vi "CRYInitialize Menu State.vi"(8 "sAction":string, 11 "Is Disable?":bool) -> ()   [LabVIEW 2013]
uses:
  SubVI/CRYMain Sub Window Global.vi
  CRYMainGlobal.vi
  CRYSystem/Task Sequence/CRYProject Run Control Global.vi
  CRYSystem/Calibration/SubVI/CRYCal Global.vi
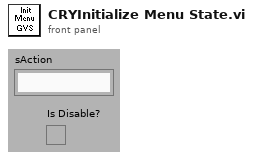
[diagram p1: front panel]
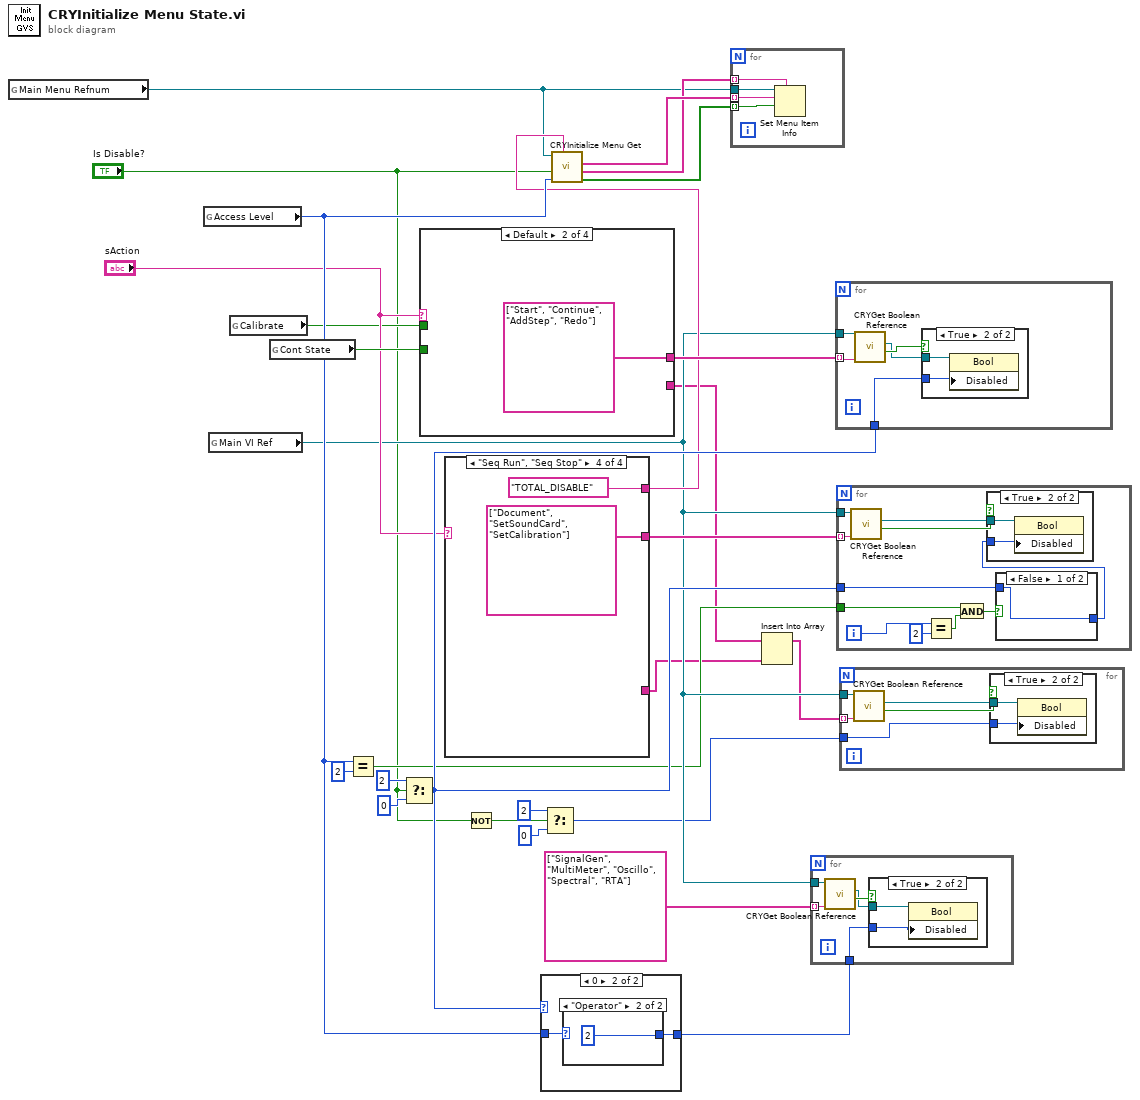
[diagram p0: block diagram]
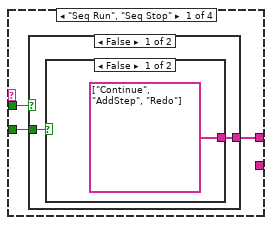
[diagram p3: hidden frame]
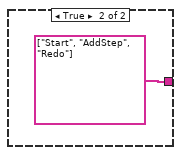
[diagram p4: hidden frame]
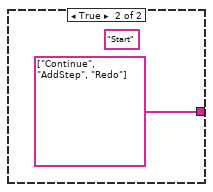
[diagram p5: hidden frame]
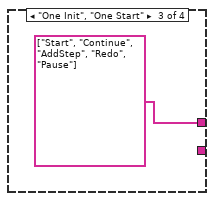
[diagram p6: hidden frame]
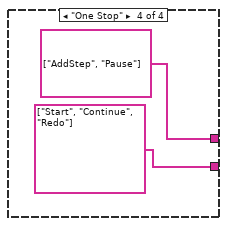
[diagram p7: hidden frame]
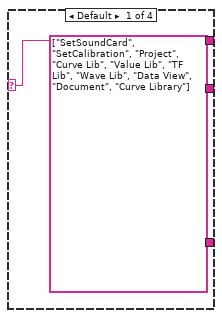
[diagram p8: hidden frame]
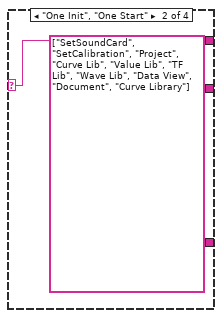
[diagram p9: hidden frame]
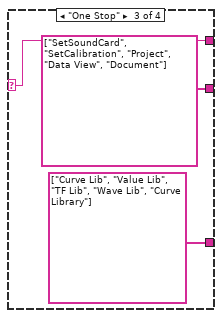
[diagram p10: hidden frame]
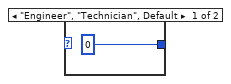
[diagram p12: hidden frame]
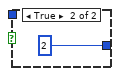
[diagram p14: hidden frame]
diagram:
  n1 = global read "CRYMain Sub Window Global.vi" "Main Menu Refnum"() -> (w1:refnum<k9>)
  n2 = global read "CRYMainGlobal.vi" "Access Level"() -> (w17:enum16{"Engineer", "Technician", "Operator"})
  n3 = global read "CRYMain Sub Window Global.vi" "Main VI Ref"() -> (w11:refnum<vi>)
  n4 = global read "CRYCal Global.vi" "Calibrate"() -> (w12:bool)
  n5 = global read "CRYProject Run Control Global.vi" "Cont State"() -> (w14:bool)
  n6 = Equal?(x=w17, y=u16 2) -> (x = y?=w10:bool)
  n7 = Select(t=u8 2 ("Disabled"), s="Is Disable?", f=u8 0) -> (s? t:f=w23:u8)
  n8 = case shown="Default" "sAction" {
    tunnel: [w29 string[] ["Start", "Continue", "AddStep", "Redo"] ("Array") string[] ["Start", "Continue", "AddStep", "Redo", "Pause"] ("Array") string[] ["AddStep", "Pause"] ("Array")] -> w26
    tunnel: w14 -> [w30 _ _ _]
    tunnel: w12 -> [w28 _ _ _]
    tunnel: [_ _ _ string[] ["Start", "Continue", "Redo"] ("Array")] -> w4
    frame "Seq Run", "Seq Stop" {
      n9 = case shown="False" w28 {
        tunnel: w30 -> [w32 _]
        tunnel: [w31 string[] ["Continue", "AddStep", "Redo"] ("Array")] -> w29
        frame False {
          n10 = case shown="False" w32 {
            tunnel: [string[] ["Continue", "AddStep", "Redo"] ("Array") string[] ["Start", "AddStep", "Redo"] ("Array")] -> w31
            frame False {
            }
            frame True {
            }
          }
        }
        frame True {
          (unwired) "Start"
        }
      }
    }
    frame Default {
    }
    frame "One Init", "One Start" {
    }
    frame "One Stop" {
    }
  }
  n11 = case shown="\"Seq Run\", \"Seq Stop\"" "sAction" {
    selector: "sAction" -> [w40 w42 w45 _]
    tunnel: [string[] ["SetSoundCard", "SetCalibration", "Project", "Curve Lib", "Value Lib", "TF Lib", "Wave Lib", "Data View", "Document", "Curve Library"] ("Array") string[] ["SetSoundCard", "SetCalibration", "Project", "Curve Lib", "Value Lib", "TF Lib", "Wave Lib", "Data View", "Document", "Curve Library"] ("Array") string[] ["SetSoundCard", "SetCalibration", "Project", "Data View", "Document"] ("Array") string[] ["Document", "SetSoundCard", "SetCalibration"] ("Array")] -> w16
    tunnel: [w40 w42 w45 "TOTAL_DISABLE"] -> w15
    tunnel: [_ _ string[] ["Curve Lib", "Value Lib", "TF Lib", "Wave Lib", "Curve Library"] ("Array") _] -> w3
    frame Default {
    }
    frame "One Init", "One Start" {
    }
    frame "One Stop" {
    }
    frame "Seq Run", "Seq Stop" {
    }
  }
  n12 = Not(x="Is Disable?") -> (.not. x?=w6:bool)
  n13 = case shown="0" w23 {
    selector: w23 -> [w49 _]
    tunnel: w17 -> [_ w51]
    tunnel: [w49 w50] -> w22
    frame Default {
    }
    frame 0 {
      n14 = case shown="\"Operator\"" w51 {
        tunnel: [u8 0 ("f") u8 2 ("Disabled")] -> w50
        frame "Engineer", "Technician", Default {
        }
        frame "Operator" {
        }
      }
    }
  }
  n15 = Select(t=u8 2 ("Disabled"), s=w6, f=u8 0) -> (s? t:f=w5:u8)
  n16 = call "CRYInitialize Menu Get.vi"("sAction"=w15, "Access Level"=w17, "Is Disable?"="Is Disable?", "Main Menu Refnum"=w1) -> ("MenuTFs"=w20:bool[], "MenuTags"=w19:string[], "MenuNames"=w21:string[])  [unwired: 5 in]
  n17 = for {
    tunnel: w21 -> [w57] mode=indexing
    tunnel: w19 -> [w56] mode=indexing
    tunnel: w20 -> [w54] mode=indexing
    tunnel: w1 -> [w55]
    n18 = Set Menu Item Info(7:w56, 9:w54, 10:w57, 11:w55) -> ()  [unwired: 1 in, 4 out]
  }
  n19 = Insert Into Array(array=w4, new element=w3) -> (w2:string[])  [unwired: 1 in]
  n20 = for {
    tunnel: w11 -> [w60]
    tunnel: w22 -> [w59]
    tunnel: string[] ["SignalGen", "MultiMeter", "Oscillo", "Spectral", "RTA"] ("Array") -> [w58] mode=indexing
    n21 = call "CRYGet Boolean Reference.vi"("Label Name"=w58, "VI Refnum"=w60) -> ("Exist?"=w62:bool, "Boolean Ref"=w61:refnum<vi>)  [unwired: 8 out]
    n22 = case shown="True" w62 {
      tunnel: w61 -> [_ w64]
      tunnel: w59 -> [_ w63]
      frame False {
      }
      frame True {
        n23 = property class="Bool"(reference=w64, "Disabled"=w63) -> ()  [unwired: 1 in, 2 out]
      }
    }
  }
  n24 = for {
    tunnel: w11 -> [w69]
    tunnel: w23 -> [w65]
    tunnel: w26 -> [w68] mode=indexing
    n25 = call "CRYGet Boolean Reference.vi"("Label Name"=w68, "VI Refnum"=w69) -> ("Exist?"=w67:bool, "Boolean Ref"=w66:refnum<vi>)  [unwired: 8 out]
    n26 = case shown="True" w67 {
      tunnel: w66 -> [_ w71]
      tunnel: w65 -> [_ w70]
      frame False {
      }
      frame True {
        n27 = property class="Bool"(reference=w71, "Disabled"=w70) -> ()  [unwired: 1 in, 2 out]
      }
    }
  }
  n28 = for {
    tunnel: w11 -> [w80]
    tunnel: w23 -> [w73]
    tunnel: w16 -> [w79] mode=indexing
    tunnel: w10 -> [w72]
    i -> [w78]
    n29 = call "CRYGet Boolean Reference.vi"("Label Name"=w79, "VI Refnum"=w80) -> ("Exist?"=w82:bool, "Boolean Ref"=w81:refnum<vi>)  [unwired: 8 out]
    n30 = Equal?(x=w78, y=2) -> (x = y?=w76:bool)
    n31 = And(x=w72, y=w76) -> (x .and. y?=w75:bool)
    n32 = case shown="False" w75 {
      tunnel: [w83 u8 2 ("f")] -> w74
      tunnel: w73 -> [w83 _]
      frame False {
      }
      frame True {
      }
    }
    n33 = case shown="True" w82 {
      tunnel: w81 -> [_ w86]
      tunnel: w74 -> [_ w85]
      frame False {
      }
      frame True {
        n34 = property class="Bool"(reference=w86, "Disabled"=w85) -> ()  [unwired: 1 in, 2 out]
      }
    }
  }
  n35 = for {
    tunnel: w11 -> [w89]
    tunnel: w5 -> [w87]
    tunnel: w2 -> [w88] mode=indexing
    n36 = call "CRYGet Boolean Reference.vi"("Label Name"=w88, "VI Refnum"=w89) -> ("Exist?"=w91:bool, "Boolean Ref"=w90:refnum<vi>)  [unwired: 8 out]
    n37 = case shown="True" w91 {
      tunnel: w90 -> [_ w93]
      tunnel: w87 -> [_ w92]
      frame False {
      }
      frame True {
        n38 = property class="Bool"(reference=w93, "Disabled"=w92) -> ()  [unwired: 1 in, 2 out]
      }
    }
  }
